vi "Spex Halt.vi"(8 "error in":errorcluster, 11 "Spex Port":refnum<visa-resource-name>) -> (0 "error out":errorcluster, 3 "Port Out":refnum<visa-resource-name>)   [LabVIEW 2010]
uses:
  <vilib>/Instr/_visa.llb/VISA Configure Serial Port (Instr).vi
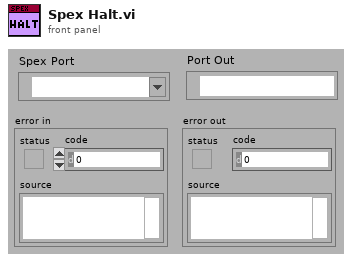
[diagram p1: front panel]
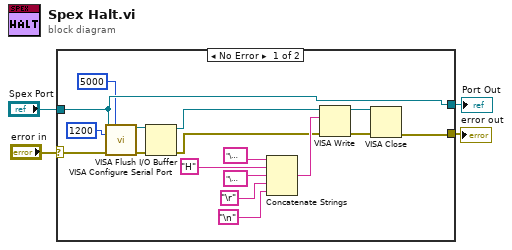
[diagram p0: block diagram]
diagram:
  n1 = case shown="No Error" "error in" {
    selector: "error in" -> [w14 w23]
    tunnel: [w9 w23] -> w4
    tunnel: [w8 w22] -> w3
    tunnel: "Spex Port" -> [w8 w22]
    frame No Error {
      n2 = call-poly "VISA Configure Serial Port"("VISA resource name"=w8, "timeout (10sec)"=u32 5000, "baud rate (9600)"=u32 1200, "error in (no error)"=w14) -> ("VISA resource name out"=w15:refnum<visa-resource-name>, "error out"=w5:errorcluster)  [unwired: 10 in]
      n3 = VISA Flush I/O Buffer(VISA resource name=w15, error in (no error)=w5) -> (VISA resource name out=w12:refnum<visa-resource-name>, error out=w13:errorcluster)  [unwired: 1 in]
      n4 = Concatenate Strings("\u0018" ("string"), "H" ("string"), "\u0003" ("string"), "\r", "\n") -> (w17:string)
      n5 = VISA Write(VISA resource name=w12, write buffer=w17, error in (no error)=w13) -> (VISA resource name out=w10:refnum<visa-resource-name>, error out=w11:errorcluster)  [unwired: 1 out]
      n6 = VISA Close(VISA resource name=w10, error in (no error)=w11) -> (error out=w9:errorcluster)
    }
    frame Error {
    }
  }
  "error out" <- w4
  "Port Out" <- w3
